vi "P_OUINON.vi"(8 "errin":errorcluster, 10 "VISAin":refnum<visa-resource-name>, 11 "Image":string) -> (0 "error out":errorcluster caption="errout", 3 "=OUI?":bool)   [LabVIEW 2020]
uses:
  <vilib>/Sylvain.lib/02 SLIM ZEN WS 500/SubVi/FGV.ctl
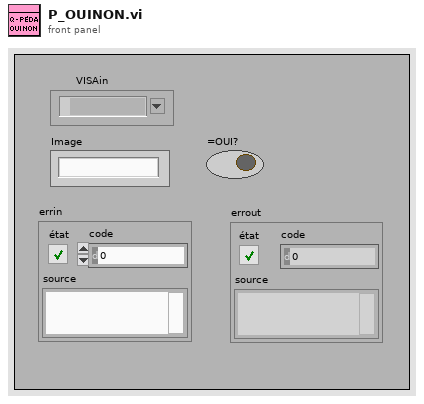
[diagram p1: front panel]
types:
  T1 = typedef "FGV.ctl" = enum16{"GET", "SET", "RAZ"}
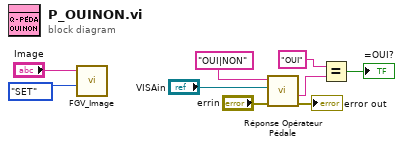
[diagram p0: block diagram]
diagram:
  n1 = call <vilib>:"FGV_Image.vi"("Énum"=FGV."SET", "IN"="Image") -> ()  [unwired: 9 in, 1 out]
  n2 = call "Réponse Opérateur Pédale.vi"("errin"="errin", "VISAin"="VISAin", "ex"="OUI|NON" ("expression régulière")) -> ("errout"=→"error out":errorcluster, "toute l'expression"=w6:string)  [unwired: 6 in, 1 out]
  n3 = Equal?(x="OUI" ("y"), y=w6) -> (x = y?=→"=OUI?":bool)
